vi "TF512 To U64x8.vi"(0 "data in":bool[](array[boolean])) -> (4 "data out":u64[](array[numeric]))   [LabVIEW 2019]
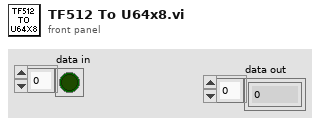
[diagram p1: front panel]
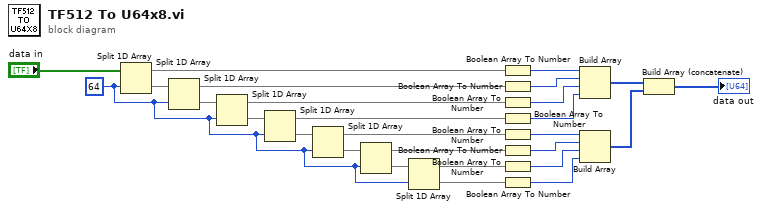
[diagram p0: block diagram]
diagram:
  w1 = 64 ("index")
  n1 = Split 1D Array(array="data in", index=w1) -> (first subarray=w20:bool[], second subarray=w2:bool[])
  n2 = Split 1D Array(array=w2, index=w1) -> (first subarray=w26:bool[], second subarray=w3:bool[])
  n3 = Split 1D Array(array=w3, index=w1) -> (first subarray=w24:bool[], second subarray=w4:bool[])
  n4 = Split 1D Array(array=w4, index=w1) -> (first subarray=w22:bool[], second subarray=w5:bool[])
  n5 = Split 1D Array(array=w5, index=w1) -> (first subarray=w15:bool[], second subarray=w6:bool[])
  n6 = Split 1D Array(array=w6, index=w1) -> (first subarray=w14:bool[], second subarray=w7:bool[])
  n7 = Split 1D Array(array=w7, index=w1) -> (first subarray=w13:bool[], second subarray=w12:bool[])
  n8 = Boolean Array To Number(Boolean array=w20) -> (number=w27:u64)
  n9 = Boolean Array To Number(Boolean array=w26) -> (number=w25:u64)
  n10 = Boolean Array To Number(Boolean array=w24) -> (number=w23:u64)
  n11 = Boolean Array To Number(Boolean array=w22) -> (number=w21:u64)
  n12 = Boolean Array To Number(Boolean array=w15) -> (number=w19:u64)
  n13 = Boolean Array To Number(Boolean array=w14) -> (number=w18:u64)
  n14 = Boolean Array To Number(Boolean array=w13) -> (number=w17:u64)
  n15 = Boolean Array To Number(Boolean array=w12) -> (number=w16:u64)
  n16 = Build Array(w27, w25, w23, w21) -> (w11:u64[])
  n17 = Build Array(w19, w18, w17, w16) -> (w9:u64[])
  n18 = Build Array (concatenate)(w11, w9) -> (→"data out":u64[])
